vi "ADCP_read_parameter.vi"(8 "error in (no error)":errorcluster, 10 "Parameter Name":string, 11 "ADCP In":refnum<class "ADCP.lvclass">) -> (0 "error out":errorcluster, 1 "Parameter Value":string, 2 "Data Packet out":T2, 3 "ADCP out":refnum<class "ADCP.lvclass">)   [LabVIEW 2017, in "ADCP.lvclass"]
uses:
  ADCP.lvclass
  ADCP_Data_Packet_Transmit_Mode.ctl
  ADCP.lvclass/ADCP.ctl
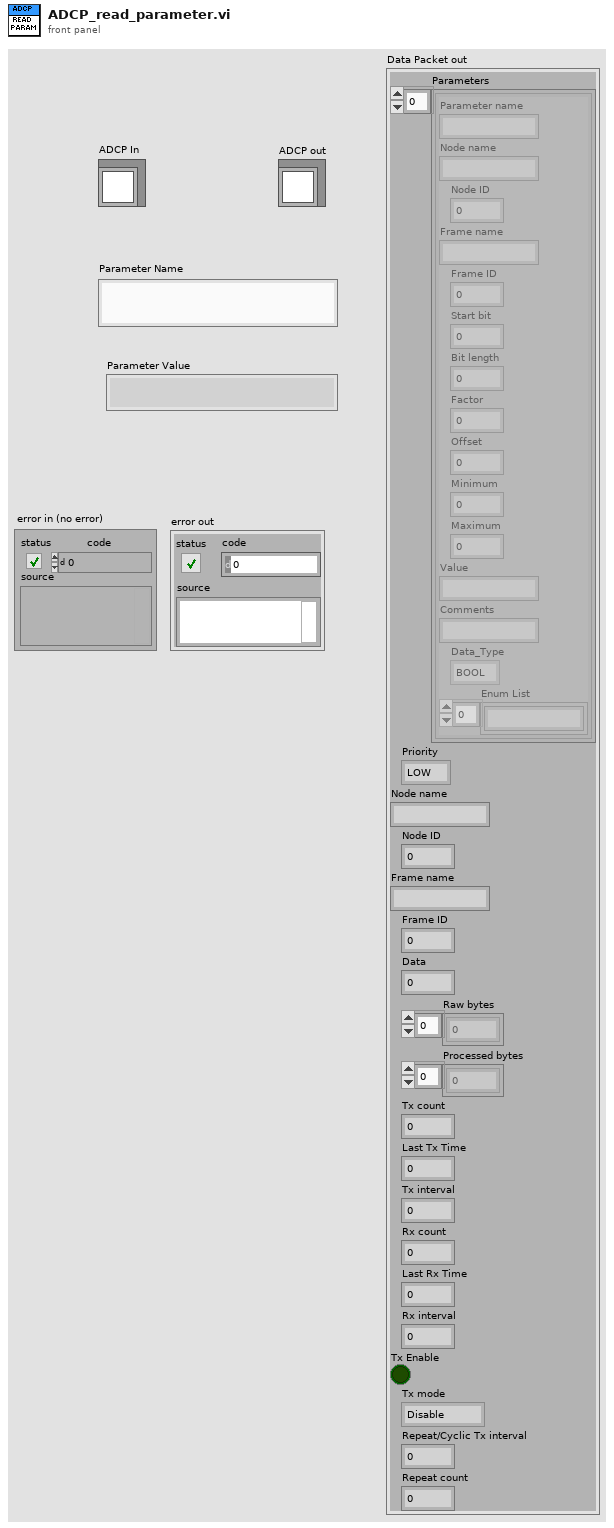
[diagram p1: front panel]
types:
  T1 = typedef "ADCP.lvclass/ADCP_Data_Packet_Transmit_Mode.ctl" = enum16{"Disable", "Single", "Cyclic", "Repeat"}
  T2 = cluster{"Parameters":cluster{"Parameter name":string, "Node name":string, "Node ID":u8, "Frame name":string, "Frame ID":u8, "Start bit":u32, "Bit length":u32, "Factor":dbl, "Offset":dbl, "Minimum":dbl, "Maximum":dbl, "Value":string, "Comments":string, "Data_Type":enum16{"BOOL", "UNSIGNED", "SIGNED", "FLOAT32", "ENUM"}, "Enum List":string[]}[], "Priority":enum16{"LOW", "HIGH"}, "Node name":string, "Node ID":u8, "Frame name":string, "Frame ID":u8, "Data":u32, "Raw bytes":u8[], "Processed bytes":u8[], "Tx count":i32, "Last Tx Time":u32, "Tx interval":u32, "Rx count":i32, "Last Rx Time":u32, "Rx interval":u32, "Tx Enable":bool, "Tx mode":T1, "Repeat/Cyclic Tx interval":u32, "Repeat count":u16}
  T3 = cluster{"Parameter name":string, "Node name":string, "Node ID":u8, "Frame name":string, "Frame ID":u8, "Start bit":u32, "Bit length":u32, "Factor":dbl, "Offset":dbl, "Minimum":dbl, "Maximum":dbl, "Value":string, "Comments":string, "Data_Type":enum16{"BOOL", "UNSIGNED", "SIGNED", "FLOAT32", "ENUM"}, "Enum List":string[]}
  T4 = enum16{"BOOL", "UNSIGNED", "SIGNED", "FLOAT32", "ENUM"}
  T5 = cluster{"Parameter name":string, "Node name":string, "Node ID":u8, "Frame name":string, "Frame ID":u8, "Start bit":u32, "Bit length":u32, "Factor":dbl, "Offset":dbl, "Minimum":dbl, "Maximum":dbl, "Value":string, "Comments":string, "Data_Type":enum16{"BOOL", "UNSIGNED", "SIGNED", "FLOAT32", "ENUM"}, "Enum List":string[]}[]
  T6 = cluster{"Parameters":cluster{"Parameter name":string, "Node name":string, "Node ID":u8, "Frame name":string, "Frame ID":u8, "Start bit":u32, "Bit length":u32, "Factor":dbl, "Offset":dbl, "Minimum":dbl, "Maximum":dbl, "Value":string, "Comments":string, "Data_Type":enum16{"BOOL", "UNSIGNED", "SIGNED", "FLOAT32", "ENUM"}, "Enum List":string[]}[], "Priority":enum16{"LOW", "HIGH"}, "Node name":string, "Node ID":u8, "Frame name":string, "Frame ID":u8, "Data":u32, "Raw bytes":u8[], "Processed bytes":u8[], "Tx count":i32, "Last Tx Time":u32, "Tx interval":u32, "Rx count":i32, "Last Rx Time":u32, "Rx interval":u32, "Tx Enable":bool, "Tx mode":T1, "Repeat/Cyclic Tx interval":u32, "Repeat count":u16}[]
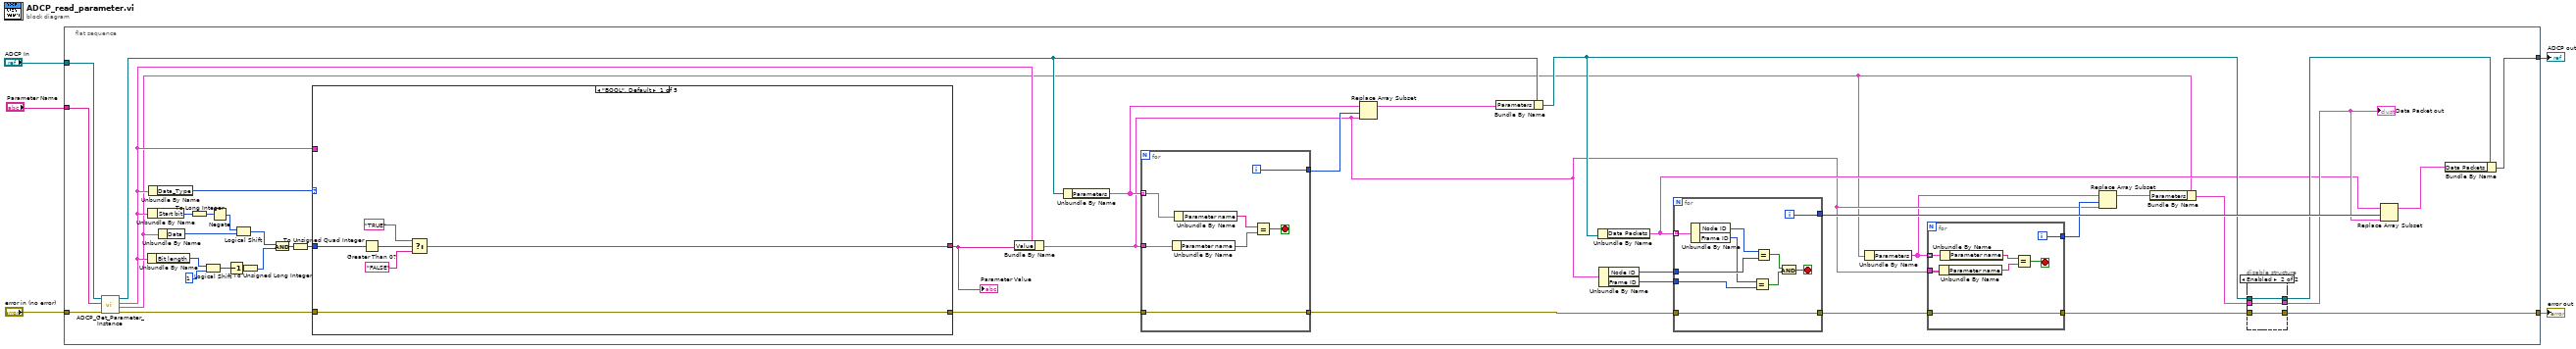
[diagram p0: block diagram]
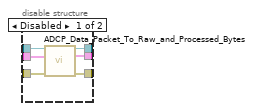
[diagram p2: hidden frame]
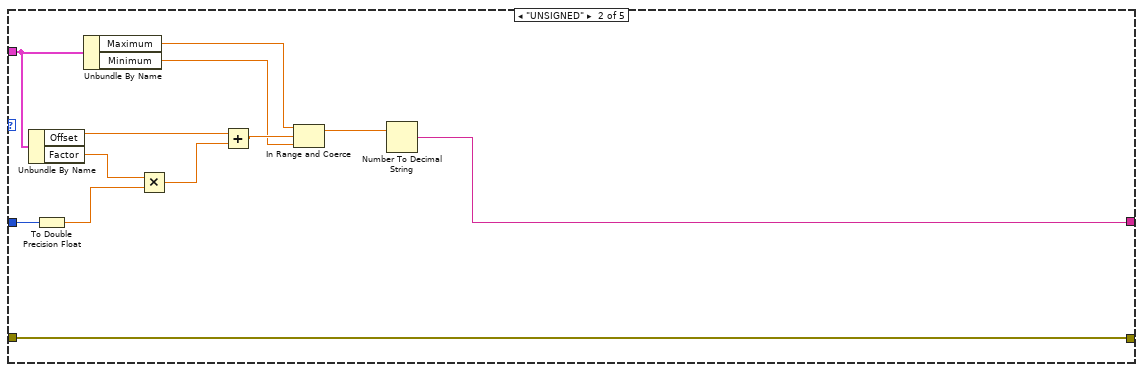
[diagram p3: hidden frame]
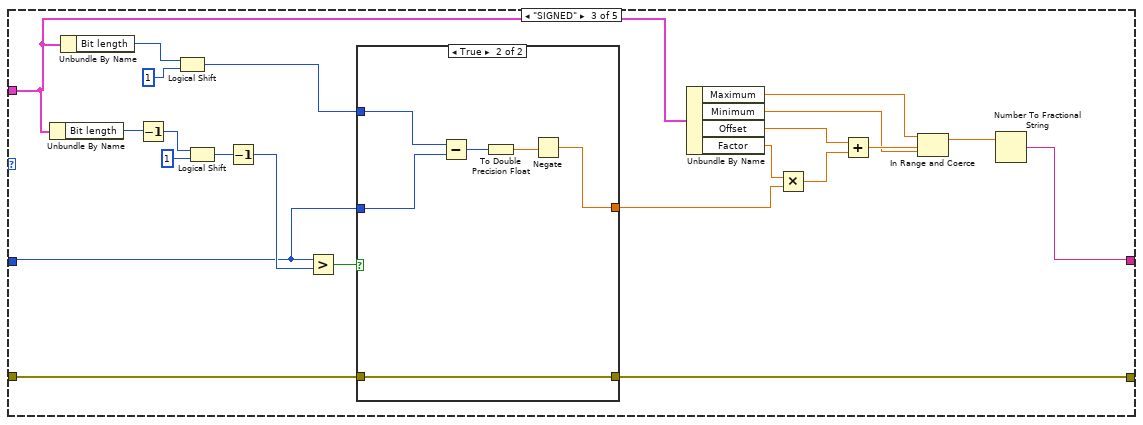
[diagram p4: hidden frame]
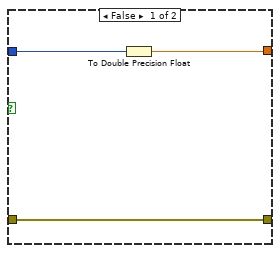
[diagram p5: hidden frame]
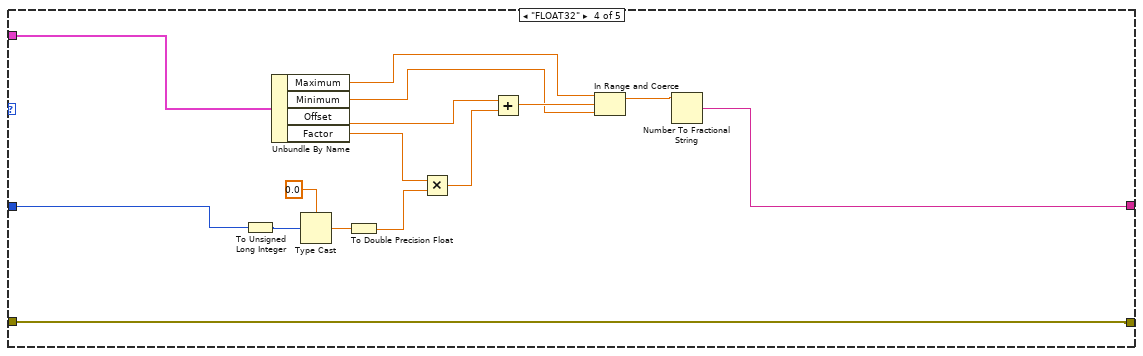
[diagram p6: hidden frame]
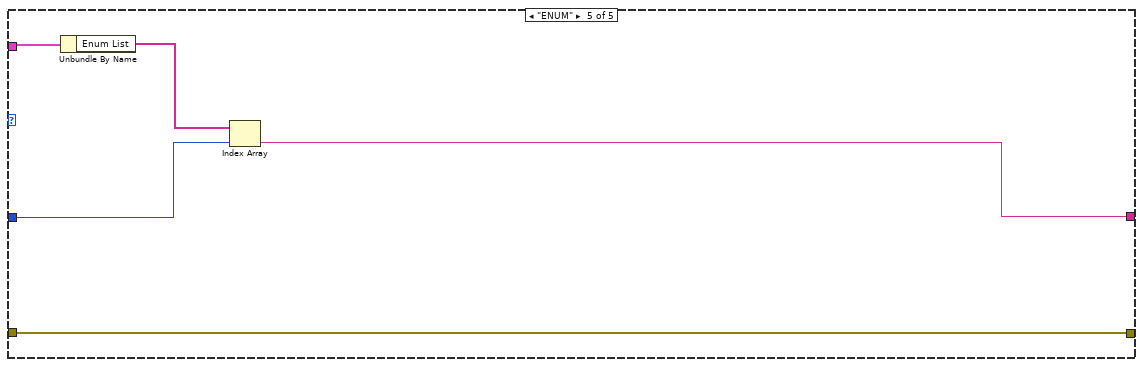
[diagram p7: hidden frame]
diagram:
  n1 = flat-sequence {
    tunnel: "ADCP In" -> [w47]
    tunnel: "Parameter Name" -> [w46]
    tunnel: "error in (no error)" -> [w48]
    tunnel: [w16] -> w2
    tunnel: [w15] -> w1
    frame #0 {
      n2 = call "ADCP_Get_Parameter_Instance.vi"("error in (no error)"=w48, "Parameter name"=w46, "ADCP in"=w47) -> ("error out"=w44:errorcluster, "Data Packet"=w8:T2, "Parameter"=w31:T3, "ADCP out"=w26:refnum<class "ADCP.lvclass">)  [unwired: 5 in]
      n3 = Unbundle By Name(w31) -> ("Bit length"=w39:u32)
      n4 = Unbundle By Name(w31) -> ("Start bit"=w42:u32)
      n5 = Unbundle By Name(w31) -> ("Data_Type"=w45:T4)
      n6 = Unbundle By Name(w8) -> ("Data"=w43:u32)
      n7 = To Long Integer(number=w42) -> (32bit integer=w41:i32)
      n8 = Logical Shift(y=w39, x=u64 1) -> (x << y=w37:u64)
      n9 = Negate(x=w41) -> (-x=w40:i32)
      n10 = Decrement(x=w37) -> (x-1=w35:u64)
      n11 = Logical Shift(y=w40, x=w43) -> (x << y=w36:u32)
      n12 = To Unsigned Long Integer(number=w35) -> (unsigned 32bit integer=w34:u32)
      n13 = And(x=w36, y=w34) -> (x .and. y?=w33:u32)
      n14 = To Unsigned Quad Integer(1:w33) -> (0:w32:u64)
      n15 = case shown="\"BOOL\", Default" w45 {
        tunnel: w44 -> [w83 w88 w116 w145 w150]
        tunnel: w32 -> [w87 w99 w114 w132 w147]
        tunnel: [w83 w88 w113 w145 w150] -> w29
        tunnel: w31 -> [_ w93 w109 w133 w149]
        tunnel: [w82 w89 w100 w131 w146] -> w30
        frame "BOOL", Default {
          n16 = Greater Than 0?(x=w87) -> (x > 0?=w86:bool)
          n17 = Select(t="TRUE", s=w86, f="FALSE") -> (s? t:f=w82:string)
        }
        frame "UNSIGNED" {
          n18 = Unbundle By Name(w93) -> ("Offset"=w95:dbl, "Factor"=w97:dbl)
          n19 = To Double Precision Float(number=w99) -> (double precision float=w98:dbl)
          n20 = Unbundle By Name(w93) -> ("Maximum"=w92:dbl, "Minimum"=w91:dbl)
          n21 = Multiply(x=w97, y=w98) -> (x*y=w96:dbl)
          n22 = Add(x=w95, y=w96) -> (x+y=w94:dbl)
          n23 = In Range and Coerce(upper limit=w92, x=w94, lower limit=w91) -> (coerced(x)=w90:dbl)  [unwired: 1 out]
          n24 = Number To Decimal String(number=w90) -> (decimal integer string=w89:string)  [unwired: 1 in]
        }
        frame "SIGNED" {
          n25 = Unbundle By Name(w109) -> ("Bit length"=w121:u32)
          n26 = Unbundle By Name(w109) -> ("Bit length"=w112:u32)
          n27 = Decrement(x=w121) -> (x-1=w120:u32)
          n28 = Logical Shift(y=w112, x=u64 1) -> (x << y=w110:u64)
          n29 = Logical Shift(y=w120, x=u64 1) -> (x << y=w118:u64)
          n30 = Decrement(x=w118) -> (x-1=w117:u64)
          n31 = Greater?(x=w114, y=w117) -> (0:w115:bool)
          n32 = case shown="True" w115 {
            tunnel: w116 -> [w123 w130]
            tunnel: w114 -> [w124 w128]
            tunnel: [w122 w125] -> w107
            tunnel: [w123 w130] -> w113
            tunnel: w110 -> [_ w129]
            frame False {
              n33 = To Double Precision Float(number=w124) -> (double precision float=w122:dbl)
            }
            frame True {
              n34 = Subtract(x=w129, y=w128) -> (x-y=w127:u64)
              n35 = To Double Precision Float(number=w127) -> (double precision float=w126:dbl)
              n36 = Negate(x=w126) -> (-x=w125:dbl)
            }
          }
          n37 = Unbundle By Name(w109) -> ("Maximum"=w103:dbl, "Minimum"=w102:dbl, "Offset"=w105:dbl, "Factor"=w108:dbl)
          n38 = Multiply(x=w108, y=w107) -> (x*y=w106:dbl)
          n39 = Add(x=w105, y=w106) -> (x+y=w104:dbl)
          n40 = In Range and Coerce(upper limit=w103, x=w104, lower limit=w102) -> (coerced(x)=w101:dbl)  [unwired: 1 out]
          n41 = Number To Fractional String(number=w101) -> (F-format string=w100:string)  [unwired: 3 in]
        }
        frame "FLOAT32" {
          n42 = To Unsigned Long Integer(number=w132) -> (unsigned 32bit integer=w144:u32)
          n43 = Unbundle By Name(w133) -> ("Maximum"=w136:dbl, "Minimum"=w135:dbl, "Offset"=w139:dbl, "Factor"=w140:dbl)
          n44 = Type Cast(type=sgl 0.0 ("single precision float"), x=w144) -> (*(type *) &x=w142:sgl)
          n45 = To Double Precision Float(number=w142) -> (double precision float=w141:dbl)
          n46 = Multiply(x=w140, y=w141) -> (x*y=w138:dbl)
          n47 = Add(x=w139, y=w138) -> (x+y=w137:dbl)
          n48 = In Range and Coerce(upper limit=w136, x=w137, lower limit=w135) -> (coerced(x)=w134:dbl)  [unwired: 1 out]
          n49 = Number To Fractional String(number=w134) -> (F-format string=w131:string)  [unwired: 3 in]
        }
        frame "ENUM" {
          n50 = Unbundle By Name(w149) -> ("Enum List"=w148:string[])
          n51 = Index Array(array=w148, index=w147) -> (element=w146:string)
        }
      }
      "Parameter Value" <- w30
      n52 = Bundle By Name(cluster=w31, "Value"=w30) -> (w11:T3)
      n53 = Unbundle By Name(w26) -> ("Parameters"=w28:T5)
      n54 = for {
        tunnel: w29 -> [w77]
        tunnel: w28 -> [w81] mode=indexing
        tunnel: w11 -> [w80]
        tunnel: [w77] -> w19
        tunnel: [w75] -> w27
        i -> [w75]
        stop <- w76 stop-if-true
        n55 = Unbundle By Name(w80) -> ("Parameter name"=w78:string)
        n56 = Unbundle By Name(w81) -> ("Parameter name"=w79:string)
        n57 = Equal?(x=w79, y=w78) -> (x = y?=w76:bool)
      }
      n58 = Replace Array Subset(array=w28, new element=w11, index=w27) -> (w25:T5)
      n59 = Bundle By Name(cluster=w26, "Parameters"=w25) -> (w18:refnum<class "ADCP.lvclass">)
      n60 = Unbundle By Name(w18) -> ("Data Packets"=w13:T6)
      n61 = Unbundle By Name(w11) -> ("Node ID"=w24:u8, "Frame ID"=w23:u8)
      n62 = for {
        tunnel: w13 -> [w65] mode=indexing
        tunnel: w24 -> [w73]
        tunnel: w23 -> [w71]
        tunnel: [w68] -> w22
        tunnel: w19 -> [w66]
        tunnel: [w66] -> w14
        i -> [w68]
        stop <- w67 stop-if-true
        n63 = Unbundle By Name(w65) -> ("Node ID"=w74:u8, "Frame ID"=w72:u8)
        n64 = Equal?(x=w72, y=w71) -> (x = y?=w69:bool)
        n65 = Equal?(x=w74, y=w73) -> (x = y?=w70:bool)
        n66 = And(x=w70, y=w69) -> (x .and. y?=w67:bool)
      }
      n67 = Unbundle By Name(w8) -> ("Parameters"=w10:T5)
      n68 = for {
        tunnel: w14 -> [w51]
        tunnel: w11 -> [w55]
        tunnel: w10 -> [w54] mode=indexing
        tunnel: [w51] -> w6
        tunnel: [w49] -> w12
        i -> [w49]
        stop <- w50 stop-if-true
        n69 = Unbundle By Name(w55) -> ("Parameter name"=w52:string)
        n70 = Unbundle By Name(w54) -> ("Parameter name"=w53:string)
        n71 = Equal?(x=w53, y=w52) -> (x = y?=w50:bool)
      }
      n72 = Replace Array Subset(array=w10, new element=w11, index=w12) -> (w9:T5)
      n73 = Bundle By Name(cluster=w8, "Parameters"=w9) -> (w7:T2)
      n74 = disable-structure shown="Enabled" {
        disable-tunnel: w6 -> [w61 w62]
        disable-tunnel: [w60 w63] -> w20
        disable-tunnel: w18 -> [w59 w64]
        disable-tunnel: [w58 w64] -> w17
        disable-tunnel: w7 -> [w57 w63]
        disable-tunnel: [w56 w62] -> w15
        frame Disabled {
          n75 = call "ADCP_Data_Packet_To_Raw_and_Processed_Bytes.vi"("ADCP In"=w59, "Data Packet In"=w57, "error in (no error)"=w61) -> ("ADCP out"=w58:refnum<class "ADCP.lvclass">, "Data Packet out"=w60:T2, "error out"=w56:errorcluster)  [unwired: 8 in, 2 out]
        }
        frame Enabled {
        }
      }
      "Data Packet out" <- w20
      n76 = Replace Array Subset(array=w13, new element=w20, index=w22) -> (w21:T6)
      n77 = Bundle By Name(cluster=w17, "Data Packets"=w21) -> (w16:refnum<class "ADCP.lvclass">)
    }
  }
  "ADCP out" <- w2
  "error out" <- w1
